vi "Check Chassis Status.vi"(8 "error in (no error)":errorcluster) -> (0 "error out":errorcluster, 1 "Chassis type Out":string, 2 "Chassis Pic Out":picture, 3 "Update?":bool)   [LabVIEW 2011]
uses:
  Controls/INIT- READ - WRITE.ctl
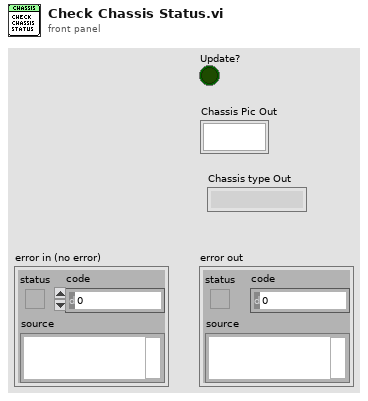
[diagram p1: front panel]
types:
  T1 = typedef "INIT- READ - WRITE.ctl" = enum16{"INIT", "READ", "WRITE"}
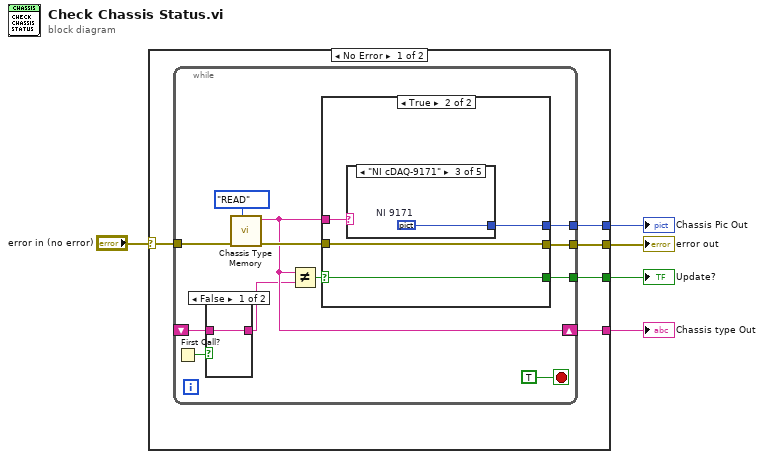
[diagram p0: block diagram]
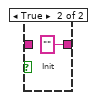
[diagram p2: hidden frame]
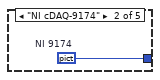
[diagram p5: hidden frame]
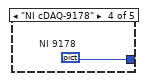
[diagram p6: hidden frame]
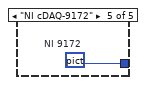
[diagram p7: hidden frame]
diagram:
  n1 = case shown="No Error" "error in (no error)" {
    selector: "error in (no error)" -> [w7 w35]
    tunnel: [w10 _] -> w5
    tunnel: [w9 w35] -> w4
    tunnel: [w8 _] -> w3
    tunnel: [w6 _] -> w1
    frame No Error {
      n2 = while {
        tunnel: w7 -> [w21]
        tunnel: [w20] -> w10
        tunnel: [w18] -> w9
        shift-right: [w15] -> w6
        shift-left: _ -> [w12]
        tunnel: [w14] -> w8
        stop <- TRUE stop-if-true
        n3 = First Call?() -> (First Call?: T/F=w13:bool)
        n4 = case shown="False" w13 {
          tunnel: w12 -> [w23 _]
          tunnel: [w23 "" ("Chassis type Out")] -> w11
          frame False {
          }
          frame True {
            # "Init"
          }
        }
        n5 = call "Chassis Type Memory.vi"("Operation"=INIT-_READ_-_WRITE."READ", "Error In"=w21) -> ("Error Out"=w19:errorcluster, "Chassis type Out"=w15:string)  [unwired: 8 in]
        n6 = Not Equal?(x=w15, y=w11) -> (x != y?=w17:bool)
        n7 = case shown="True" w17 {
          selector: w17 -> [w25 w27]
          tunnel: w15 -> [_ w30]
          tunnel: [_ w29] -> w20
          tunnel: w19 -> [w26 w28]
          tunnel: [w26 w28] -> w18
          tunnel: [w25 w27] -> w14
          frame False {
          }
          frame True {
            n8 = case shown="\"NI cDAQ-9171\"" w30 {
              tunnel: [_ w31 w32 w33 w34] -> w29
              frame Default {
              }
              frame "NI cDAQ-9174" {
                w31 = picture bytes[792642]  # NI 9174
              }
              frame "NI cDAQ-9171" {
                w32 = picture bytes[774678]  # NI 9171
              }
              frame "NI cDAQ-9178" {
                w33 = picture bytes[770502]  # NI 9178
              }
              frame "NI cDAQ-9172" {
                w34 = picture bytes[774678]  # NI 9172
              }
            }
          }
        }
      }
    }
    frame Error {
    }
  }
  "error out" <- w4
  "Chassis Pic Out" <- w5
  "Update?" <- w3
  "Chassis type Out" <- w1
